vi "CountAtoms.vi"(9 "Background Image":dbl[][](graph), 10 "Atom Image":dbl[][](graph), 11 "Cursor List":T1) -> (1 "Number":dbl, 2 "OD":dbl[][](graph))   [LabVIEW 2013]
uses:
  <vilib>/Utility/miscctls.llb/LVCursorListTypeDef.ctl
  <vilib>/Utility/file.llb/Write To Spreadsheet File (DBL).vi
  <vilib>/Utility/file.llb/Read From Spreadsheet File (DBL).vi
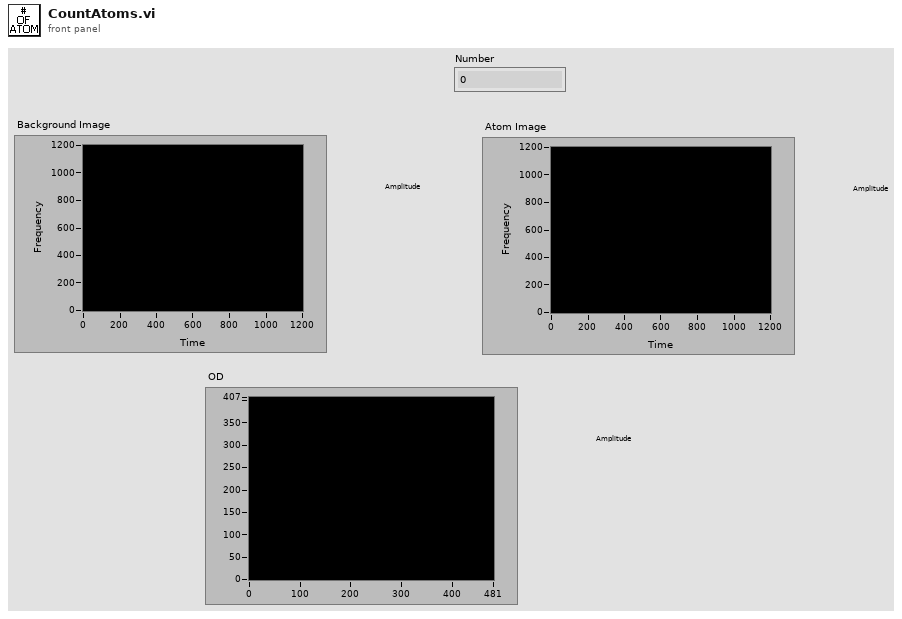
[diagram p1: front panel]
types:
  T1 = typedef "LVCursorListTypeDef.ctl" = cluster{"Name":string, "Color":u32, "Style":u8, "Point Style":u8, "Name Visible":bool, "Allow Drag":bool, "Cursor Mode":u32, "Plot":i32, "Index":i32, "Position":cluster{"X":dbl, "Y":dbl}, "X Scale":u32, "Y Scale":u32, "Watch Plots":i32[], "Watch All Plots":bool, "Plot Area":i32, "Label Offset":cluster{"X":dbl, "Y":dbl}}[]
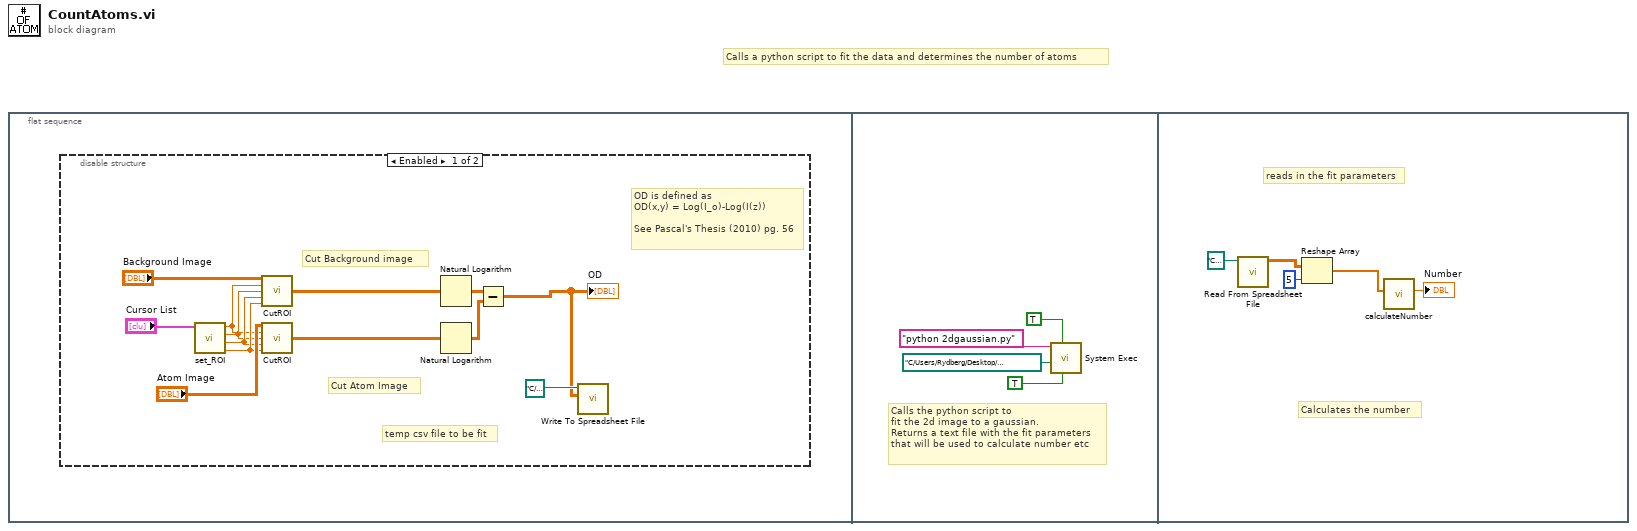
[diagram p0: block diagram]
diagram:
  # "Calls a python script to fit the data and determines the number of atoms"
  n1 = flat-sequence {
    frame #0 {
      n2 = disable-structure shown="Enabled" {
        frame Enabled {
          # "temp csv file to be fit"
          # "OD is defined as \nOD(x,y) = Log(I_o)-Log(I(z))\n\nSee Pascal's Thesis (2010) pg. 56"
          # "Cut Atom Image"
          # "Cut Background image"
          n3 = call "set_ROI.vi"("Cursor List"="Cursor List") -> ("Row End"=w6:dbl, "RowStart"=w5:dbl, "ColEnd"=w4:dbl, "ColStart"=w3:dbl)  [unwired: 7 in]
          n4 = call "CutROI.vi"("Full Image In"="Background Image", "Col Start"=w3, "Col End"=w4, "Row Start"=w5, "Row End"=w6) -> ("Cut Image Out"=w10:dbl[][])  [unwired: 10 in]
          n5 = call "CutROI.vi"("Full Image In"="Atom Image", "Col Start"=w3, "Col End"=w4, "Row Start"=w5, "Row End"=w6) -> ("Cut Image Out"=w9:dbl[][])  [unwired: 10 in]
          n6 = Natural Logarithm(1:w10) -> (0:w8:dbl[][])
          n7 = Natural Logarithm(1:w9) -> (0:w7:dbl[][])
          n8 = Subtract(x=w8, y=w7) -> (x-y=w1:dbl[][])
          "OD" <- w1
          n9 = call-poly <vilib>:"Write To Spreadsheet File.vi"("2D data"=w1, "file path (dialog if empty)"=path "C:/Users/Rydberg/Desktop/JoeDesktopFiles/LabView/testing ground/RydbergExpControl/temp.csv") -> ()  [unwired: 6 in, 1 out]
        }
        frame Disabled {
        }
      }
    }
    frame #1 {
      # "Calls the python script to\nfit the 2d image to a gaussian.\nReturns a text file with the fit parameters\nthat will be used to calculate number etc"
      n10 = call <vilib>:"System Exec.vi"("run minimized? (F)"=TRUE, "wait until completion? (T)"=TRUE, "working directory"=path "C:/Users/Rydberg/Desktop/JoeDesktopFiles/LabView/testing ground/RydbergExpControl", "command line"="python 2dgaussian.py") -> ()  [unwired: 4 in, 4 out]
    }
    frame #2 {
      # "Calculates the number"
      # "reads in the fit parameters"
      n11 = call-poly <vilib>:"Read From Spreadsheet File.vi"("file path (dialog if empty)"=path "C:/Users/Rydberg/Desktop/JoeDesktopFiles/LabView/testing ground/RydbergExpControl/fitparams.txt") -> ("all rows"=w21:dbl[][])  [unwired: 6 in, 4 out]
      n12 = Reshape Array(w21, 5 ("dimension size")) -> (w19:dbl[])
      n13 = call "calculateNumber.vi"("Array"=w19) -> ("Number"=→"Number":dbl)  [unwired: 10 in]
    }
  }
